vi "global-2.vi"() -> ()   [LabVIEW 2015]
panel:
  in  "开入":T1
  out "软压板R":T2 caption="继保遥信"
  out "动作报告":T3
  out "虚遥信":T4
  out "遥控R":bool[](array[boolean])
  out "遥测":u32[](array[numeric])
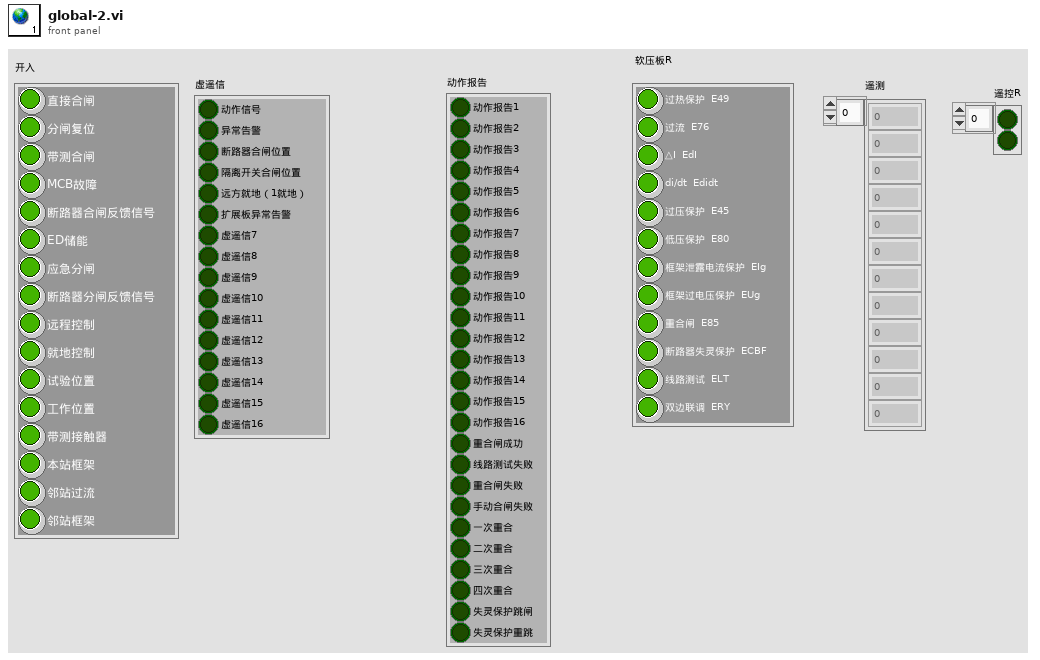
[diagram p1: front panel]
types:
  T1 = cluster{"直接合闸":bool, "分闸复位":bool, "带测合闸":bool, "MCB故障":bool, "断路器合闸反馈信号":bool, "ED储能":bool, "应急分闸":bool, "断路器分闸反馈信号":bool, "远程控制":bool, "就地控制":bool, "试验位置":bool, "工作位置":bool, "带测接触器":bool, "本站框架":bool, "邻站过流":bool, "邻站框架":bool}
  T2 = cluster{"过热保护  E49":bool, "过流  E76":bool, "△I  EdI":bool, "di/dt  Edidt":bool, "过压保护  E45":bool, "低压保护  E80":bool, "框架泄露电流保护  EIg":bool, "框架过电压保护  EUg":bool, "重合闸  E85":bool, "断路器失灵保护  ECBF":bool, "线路测试  ELT":bool, "双边联调  ERY":bool}
  T3 = cluster{"动作报告1":bool, "动作报告2":bool, "动作报告3":bool, "动作报告4":bool, "动作报告5":bool, "动作报告6":bool, "动作报告7":bool, "动作报告8":bool, "动作报告9":bool, "动作报告10":bool, "动作报告11":bool, "动作报告12":bool, "动作报告13":bool, "动作报告14":bool, "动作报告15":bool, "动作报告16":bool, "重合闸成功":bool, "线路测试失败":bool, "重合闸失败":bool, "手动合闸失败":bool, "一次重合":bool, "二次重合":bool, "三次重合":bool, "四次重合":bool, "失灵保护跳闸":bool, "失灵保护重跳":bool}
  T4 = cluster{"动作信号":bool, "异常告警":bool, "断路器合闸位置":bool, "隔离开关合闸位置":bool, "远方就地（1就地）":bool, "扩展板异常告警":bool, "虚遥信7":bool, "虚遥信8":bool, "虚遥信9":bool, "虚遥信10":bool, "虚遥信11":bool, "虚遥信12":bool, "虚遥信13":bool, "虚遥信14":bool, "虚遥信15":bool, "虚遥信16":bool}
diagram:
